vi "Global.vi"() -> ()   [LabVIEW 2022 SP3]
uses:
  Control 1.ctl
panel:
  out "Encoding Checksum":T1
  out "Decoding Checksum":string
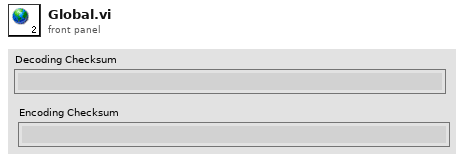
[diagram p1: front panel]
types:
  T1 = typedef "Control 1.ctl" = string
diagram:
